vi "Process Acknowledgement.vi"(8 "error in (no error)":errorcluster, 10 "Incoming Packet":refnum<class "ControlPacket.lvclass">, 11 "Session in":refnum<class "Session.lvclass">) -> (0 "error out":errorcluster, 3 "Session out":refnum<class "Session.lvclass">)   [LabVIEW 2013, in "MQTT Base.lvlib" / "Session.lvclass"]
uses:
  Session.lvclass
  <vilib>/LabVIEW Open Source Project/MQTT Control Packets/Control Packets/ControlPacket/ControlPacket.lvclass
  Session.lvclass/Session.ctl
  Base Class/Response -- cluster.ctl
  Base Class/MQTT_Base.lvclass
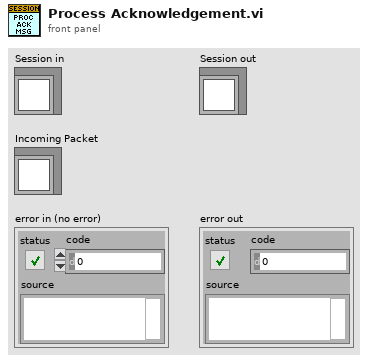
[diagram p1: front panel]
types:
  T1 = typedef "MQTT Base.lvlib/MQTT_Base.lvclass/Response -- cluster.ctl" = cluster{"Packet":refnum<class "ControlPacket.lvclass">, "Protocol Error":errorcluster, "disconnect session":bool, "[ACK]":refnum<notifier>[]}
  T2 = typedef "MQTT Base.lvlib/Session.lvclass/Pending ACKs -- cluster.ctl" = cluster{"Message":refnum<class "ControlPacket.lvclass">, "[ACK]":refnum<notifier>[], "Packet Identifier":u32}
  T3 = typedef "MQTT Base.lvlib/Session.lvclass/Session State -- cluster.ctl" = cluster{"CleanSession":bool, "Client ID":string, "Subscriptions":T4[], "Pending Transmissions":T6[], "Pending ACKs":T2[], "Pending ACK map":variant}
  T4 = typedef "MQTT_Control_Packets.lvlib/SUBSCRIBE.lvclass/Topic Subscription -- cluster.ctl" = cluster{"Topic Filter":string, "QoS":T5}
  T5 = typedef "MQTT_Control_Packets.lvlib/ControlPacket.lvclass/QualityOfService -- enum.ctl" = enum16{"0 (At Most Once)", "1 (At Least Once)", "2 (Exactly Once)"}
  T6 = typedef "MQTT_Control_Packets.lvlib/ControlPacket.lvclass/Pending Transmission -- cluster.ctl" = cluster{"Message":refnum<class "ControlPacket.lvclass">, "QoS":T5, "Tx-Rx":bool}
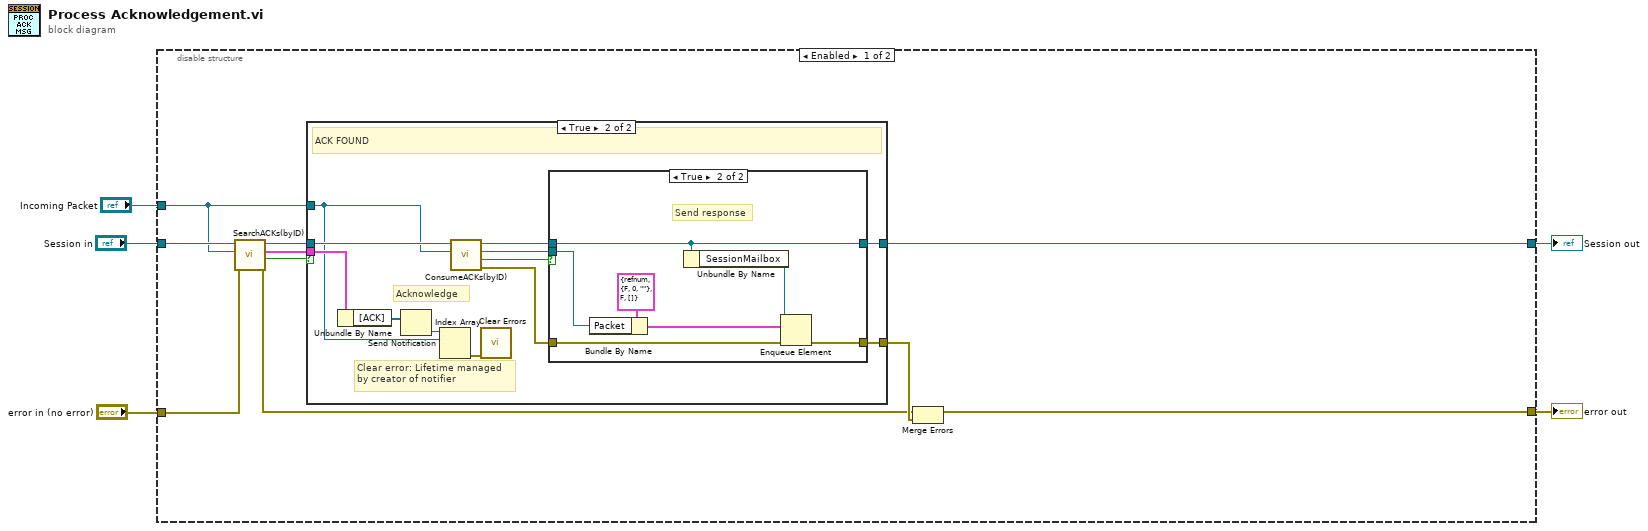
[diagram p0: block diagram]
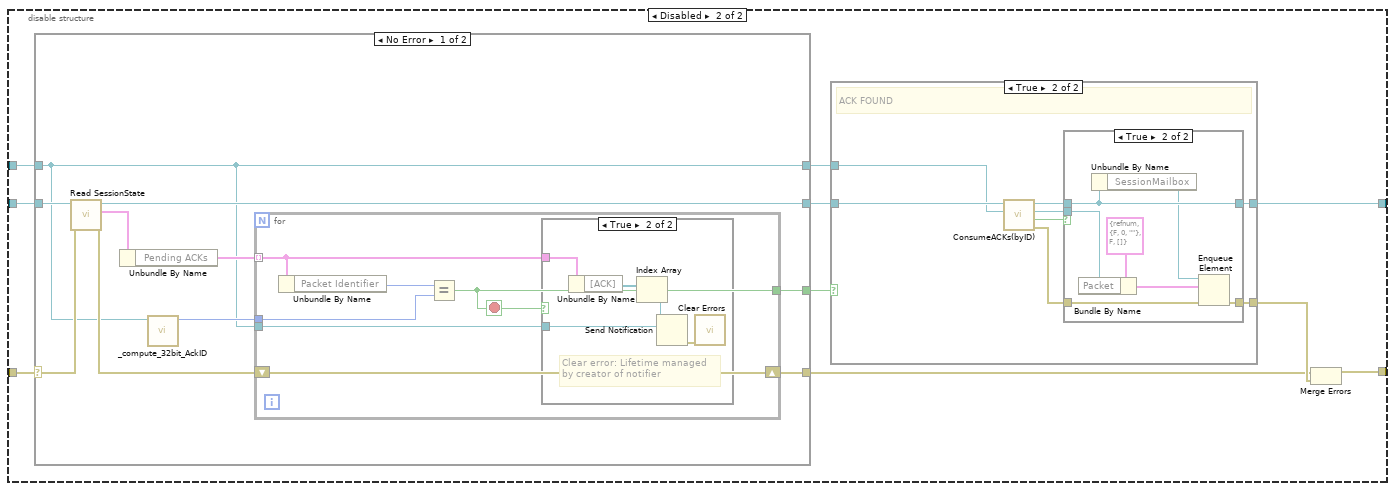
[diagram p4: hidden frame]
diagram:
  n1 = disable-structure shown="Enabled" {
    disable-tunnel: "Incoming Packet" -> [w6 w38]
    disable-tunnel: "error in (no error)" -> [w10 w40]
    disable-tunnel: "Session in" -> [w9 w44]
    disable-tunnel: [w8 w46] -> w2
    disable-tunnel: [w7 w45] -> w1
    frame Enabled {
      n2 = call "SearchACKs(byID).vi"("error in (no error)"=w10, "ControlPacket in"=w6, "Session in"=w9) -> ("error out"=w14:errorcluster, "found?"=w11:bool, "Pending ACK"=w12:T2, "Session out"=w13:refnum<class "Session.lvclass">)  [unwired: 5 in]
      n3 = case shown="True" w11 {
        tunnel: w12 -> [_ w25]
        tunnel: w13 -> [w16 w24]
        tunnel: [w16 w23] -> w8
        tunnel: w6 -> [_ w19]
        tunnel: [_ w22] -> w15
        frame False {
        }
        frame True {
          # "Acknowledge"
          # "Clear error: Lifetime managed\nby creator of notifier"
          # "ACK FOUND"
          n4 = Unbundle By Name(w25) -> ("[ACK]"=w28:refnum<notifier>[])
          n5 = Index Array(array=w28) -> (element=w27:refnum<notifier>)  [unwired: 1 in]
          n6 = Send Notification(notification=w19, notifier=w27) -> (error out=w26:errorcluster)  [unwired: 1 in, 1 out]
          n7 = call "ConsumeACKs(byID).vi"("ControlPacket in"=w19, "Session in"=w24) -> ("error out"=w20:errorcluster, "response prepared?"=w17:bool, "ControlPacket response"=w18:refnum<class "ControlPacket.lvclass">, "Session out"=w21:refnum<class "Session.lvclass">)  [unwired: 6 in]
          n8 = call <vilib>:"Clear Errors.vi"("error in (no error)"=w26) -> ()  [unwired: 6 in, 1 out]
          n9 = case shown="True" w17 {
            tunnel: w21 -> [w30 w32]
            tunnel: [w29 w35] -> w22
            tunnel: [w30 w32] -> w23
            tunnel: w18 -> [_ w34]
            tunnel: w20 -> [w29 w33]
            frame False {
            }
            frame True {
              # "Send response"
              n10 = Bundle By Name(cluster=T1 {"Packet"=refnum, "Protocol Error"={"status"=FALSE, "code"=0, "source"=""}, "disconnect session"=FALSE, "[ACK]"=[]} ("element"), "Packet"=w34) -> (w36:T1)
              n11 = Unbundle By Name(w32) -> ("SessionMailbox"=w31:refnum<queue>)
              n12 = Enqueue Element(queue=w31, element=w36, error in (no error)=w33) -> (error out=w35:errorcluster)  [unwired: 1 in, 2 out]
            }
          }
        }
      }
      n13 = Merge Errors(w14, w15) -> (w7:errorcluster)
    }
    frame Disabled {
      n14 = case shown="No Error" w40 {
        selector: w40 -> [w54 w70]
        tunnel: [w49 w70] -> w41
        tunnel: [w51 w71] -> w43
        tunnel: w44 -> [w52 w71]
        tunnel: [w55 _] -> w42
        tunnel: w38 -> [w48 w69]
        tunnel: [w48 w69] -> w39
        frame No Error {
          n15 = call "Read SessionState.vi"("error in (no error)"=w54, "Session in"=w52) -> ("error out"=w50:errorcluster, "Session State"=w57:T3, "Session out"=w51:refnum<class "Session.lvclass">)  [unwired: 7 in]
          n16 = Unbundle By Name(w57) -> ("Pending ACKs"=w56:T2[])
          n17 = call "_compute_32bit_AckID.vi"("ControlPacket in"=w48) -> ("ACK ID"=w53:u32)  [unwired: 10 in]
          n18 = for {
            tunnel: w56 -> [w59] mode=indexing
            tunnel: [w60] -> w55
            tunnel: w53 -> [w62]
            shift-right: [w61] -> w49
            shift-left: w50 -> [w61]
            tunnel: w48 -> [w58]
            stop <- w60 stop-if-true
            n19 = Unbundle By Name(w59) -> ("Packet Identifier"=w63:u32)
            n20 = Equal?(x=w63, y=w62) -> (x = y?=w60:bool)
            n21 = case shown="True" w60 {
              tunnel: w59 -> [_ w68]
              tunnel: w58 -> [_ w65]
              frame False {
              }
              frame True {
                # "Clear error: Lifetime managed\nby creator of notifier"
                n22 = Unbundle By Name(w68) -> ("[ACK]"=w67:refnum<notifier>[])
                n23 = Index Array(array=w67) -> (element=w66:refnum<notifier>)  [unwired: 1 in]
                n24 = Send Notification(notification=w65, notifier=w66) -> (error out=w64:errorcluster)  [unwired: 1 in, 1 out]
                n25 = call <vilib>:"Clear Errors.vi"("error in (no error)"=w64) -> ()  [unwired: 6 in, 1 out]
              }
            }
          }
        }
        frame Error {
        }
      }
      n26 = case shown="True" w42 {
        tunnel: w43 -> [w72 w80]
        tunnel: [w72 w79] -> w46
        tunnel: w39 -> [_ w75]
        tunnel: [_ w78] -> w47
        frame False {
        }
        frame True {
          # "ACK FOUND"
          n27 = call "ConsumeACKs(byID).vi"("ControlPacket in"=w75, "Session in"=w80) -> ("error out"=w76:errorcluster, "response prepared?"=w73:bool, "ControlPacket response"=w74:refnum<class "ControlPacket.lvclass">, "Session out"=w77:refnum<class "Session.lvclass">)  [unwired: 6 in]
          n28 = case shown="True" w73 {
            tunnel: w77 -> [w82 w84]
            tunnel: [w81 w87] -> w78
            tunnel: [w82 w84] -> w79
            tunnel: w74 -> [_ w86]
            tunnel: w76 -> [w81 w85]
            frame False {
            }
            frame True {
              n29 = Bundle By Name(cluster=T1 {"Packet"=refnum, "Protocol Error"={"status"=FALSE, "code"=0, "source"=""}, "disconnect session"=FALSE, "[ACK]"=[]} ("element"), "Packet"=w86) -> (w88:T1)
              n30 = Unbundle By Name(w84) -> ("SessionMailbox"=w83:refnum<queue>)
              n31 = Enqueue Element(queue=w83, element=w88, error in (no error)=w85) -> (error out=w87:errorcluster)  [unwired: 1 in, 2 out]
            }
          }
        }
      }
      n32 = Merge Errors(w41, w47) -> (w45:errorcluster)
    }
  }
  "Session out" <- w2
  "error out" <- w1
